vi "Request Check-out Details.vi"(0 "Hotel Management Tool Model in":refnum<class "Hotel Management Tool Model.lvclass">, 5 "Rooms Manager GUID":string, 7 "Room No":string, 11 "error in (no error)":errorcluster) -> (4 "Hotel Management Tool Model out":refnum<class "Hotel Management Tool Model.lvclass">, 15 "error out":errorcluster)   [LabVIEW 2023, in "Hotel Management Tool Model.lvlib" / "Hotel Management Tool Model.lvclass"]
uses:
  Hotel Management Tool Model.lvclass
  Hotel Management Tool Model.lvclass/Hotel Management Tool Model.ctl
  Central Data Manager/Central Data Manager Messages/Fetch Check-out Details Msg/Fetch Check-out Details Msg.lvclass/Fetch Check-out Details Msg.ctl
  <vilib>/ActorFramework/Message Enqueuer/Message Enqueuer.lvclass/Message Enqueuer.ctl
  <vilib>/ActorFramework/Message Enqueuer/Enqueue.vi
  Central Data Manager/Central Data Manager Messages/Fetch Check-out Details Msg/Fetch Check-out Details Msg.lvclass
  C:/Program Files/National Instruments/LabVIEW 2023/vi.lib/ActorFramework/Message/Message.lvclass
  <vilib>/ActorFramework/Stop Msg/Stop Msg.lvclass
  <vilib>/ActorFramework/Message Priority Queue/Priority Enqueue.vi
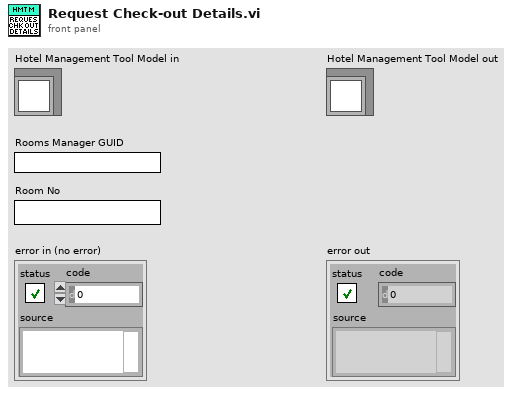
[diagram p1: front panel]
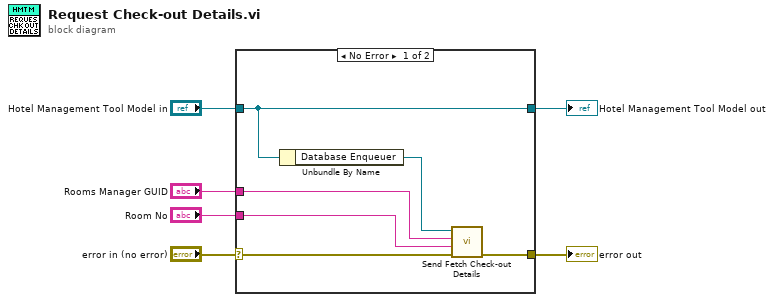
[diagram p0: block diagram]
diagram:
  n1 = case shown="No Error" "error in (no error)" {
    selector: "error in (no error)" -> [w9 w14]
    tunnel: [w7 w14] -> w4
    tunnel: [w12 w13] -> w6
    tunnel: "Hotel Management Tool Model in" -> [w12 w13]
    tunnel: "Rooms Manager GUID" -> [w10 _]
    tunnel: "Room No" -> [w8 _]
    frame No Error {
      n2 = Unbundle By Name(w12) -> ("Database Enqueuer"=w11:refnum<class "Message Enqueuer.lvclass">)
      n3 = call "Send Fetch Check-out Details.vi"("error in (no error)"=w9, "Room No"=w8, "Rooms Manager GUID"=w10, "Message Enqueuer"=w11) -> ("error out"=w7:errorcluster)  [unwired: 6 in, 1 out]
    }
    frame Error {
    }
  }
  "error out" <- w4
  "Hotel Management Tool Model out" <- w6
